vi "LDT Parse XML Time.vi"(8 "error in (no error)":errorcluster, 11 "Time String":string="   <time>2020-09-14T20:44:15.228+00:00</time>\n") -> (0 "error out":errorcluster, 2 "Time string":string)   [LabVIEW 2022 SP3, in "LDT Telescope.lvclass"]
uses:
  LDT Telescope.lvclass
panel:
  out "time stamp":timestamp
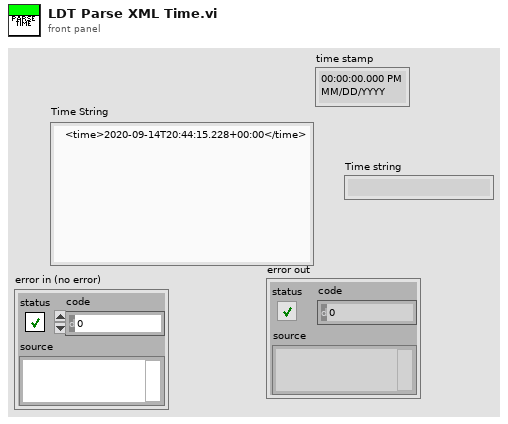
[diagram p1: front panel]
types:
  T1 = typedef "LVDateTimeRec.ctl" = cluster{"fractional second":dbl, "second":i32, "minute":i32, "hour":i32, "day of month":i32, "month":i32, "year":i32, "day of week":i32, "day of year":i32, "DST":i32}
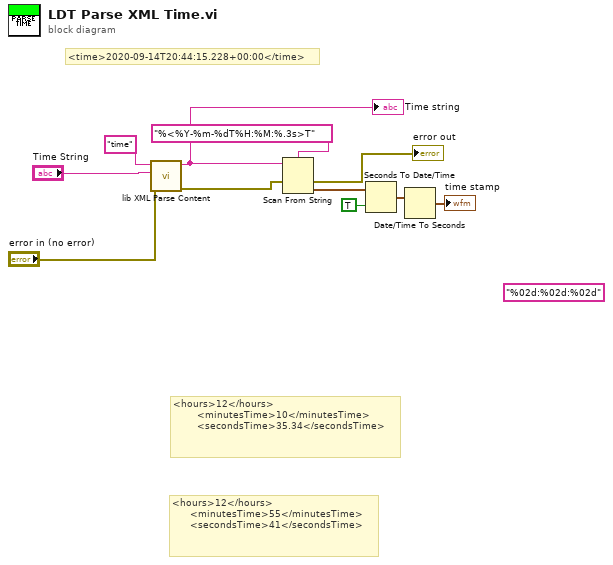
[diagram p0: block diagram]
diagram:
  (unwired) "%02d:%02d:%02d" ("format string")
  # "<time>2020-09-14T20:44:15.228+00:00</time>"
  # "<hours>12</hours>\n      <minutesTime>55</minutesTime>\n      <secondsTime>41</secondsTime>"
  # "<hours>12</hours>\n        <minutesTime>10</minutesTime>\n        <secondsTime>35.34</secondsTime>"
  n1 = call "lib XML Parse Content.vi"("error in (no error)"="error in (no error)", "XML Line"="Time String", "XML Topic"="time") -> ("error out"=w2:errorcluster, "Content"=w3:string)  [unwired: 6 in, 1 out]
  "Time string" <- w3
  n2 = Scan From String(format string="%<%Y-%m-%dT%H:%M:%.3s>T", input string=w3, error in=w2) -> (error out=→"error out":errorcluster, output 1=w6:timestamp)  [unwired: 2 in, 2 out]
  n3 = Seconds To Date/Time(time stamp (now)=w6, to UTC (F)=TRUE) -> (date time rec=w7:T1)
  n4 = Date/Time To Seconds(2:w7) -> (0:→"time stamp":timestamp)  [unwired: 1 in]
